vi "check_empty_path.vi"(8 "error in":errorcluster, 11 "Path to check":path) -> (0 "error out":errorcluster, 3 "Path to check out":path)   [LabVIEW 2019]
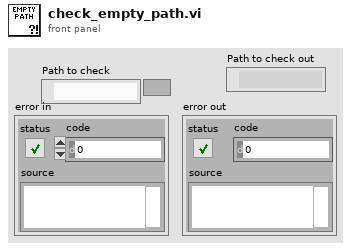
[diagram p1: front panel]
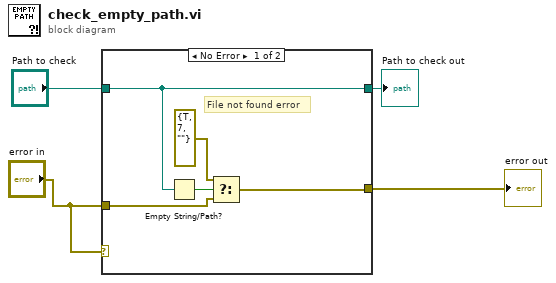
[diagram p0: block diagram]
diagram:
  n1 = case shown="No Error" "error in" {
    tunnel: [w9 w11] -> w4
    tunnel: "Path to check" -> [w5 w10]
    tunnel: "error in" -> [w6 w11]
    tunnel: [w5 w10] -> w1
    frame No Error {
      # "File not found error"
      n2 = Empty String/Path?(string/path=w5) -> (empty?=w7:bool)
      n3 = Select(t=errorcluster {"status"=TRUE, "code"=7, "source"=""} ("error constant"), s=w7, f=w6) -> (s? t:f=w9:errorcluster)
    }
    frame Error {
    }
  }
  "error out" <- w4
  "Path to check out" <- w1
